vi "SET Log Ref.vi"(8 "error in (no error)":errorcluster, 11 "LogsAbstract in":refnum<class "LogsAbstract.lvclass">) -> (0 "error out":errorcluster, 3 "LogsAbstract out":refnum<class "LogsAbstract.lvclass">)   [LabVIEW 2019, in "LogsAbstract.lvlib" / "LogsAbstract.lvclass"]
uses:
  LogsAbstract.lvclass
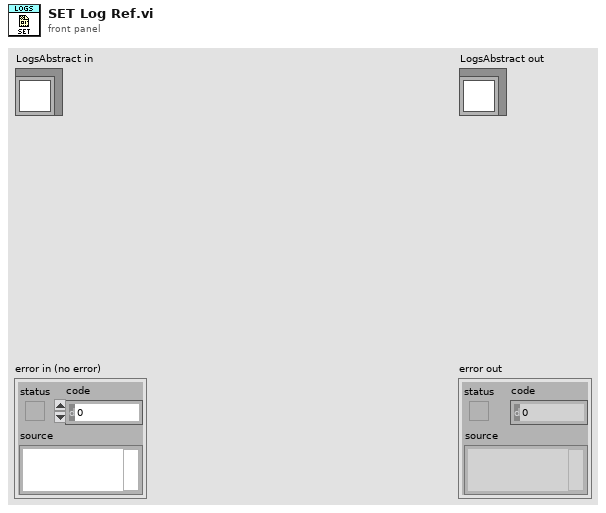
[diagram p1: front panel]
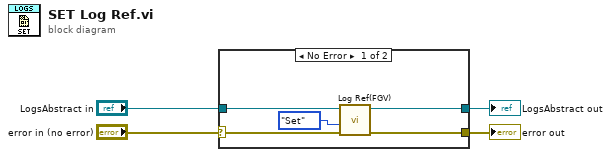
[diagram p0: block diagram]
diagram:
  n1 = case shown="No Error" "error in (no error)" {
    selector: "error in (no error)" -> [w7 w11]
    tunnel: [w6 w11] -> w3
    tunnel: [w8 w10] -> w1
    tunnel: "LogsAbstract in" -> [w9 w10]
    frame No Error {
      n2 = call-dynamic "Log Ref(FGV).vi"("Error In"=w7, "State"=enum16{"Get", "Set"}."Set", "EventLog In"=w9) -> ("Error Out"=w6:errorcluster, "EventLog Out"=w8:refnum<class "LogsAbstract.lvclass">)  [unwired: 7 in]
    }
    frame Error {
    }
  }
  "error out" <- w3
  "LogsAbstract out" <- w1
